vi "PID Online Autotuning (PID on the loop).vi"(0 "setpoint":dbl(slide)=30.8641975308642 scale=0.0..100.0 scale format="%.1f", 1 "manipulated variable":dbl, 3 "autotuning parameters":T2={"type of controller"=1, "relay cycles"=3, "relay amplitude"=1.0, "control specifications"=2, "PV noise level"=0.1} {"PV noise level" format="%.2f"; "control specifications" items=["Fast", "Normal", "Slow"]; "relay amplitude" format="%.2f"; "type of controller" items=["P", "PI", "PID"]}, 5 "process variable":dbl(slide)=19.583333333333336 scale=0.0..100.0 scale format="%.1f", 9 "PID gains in":T1={"proportional gain (Kc)"=1.0, "integral time (Ti, min)"=0.01, "derivative time (Td, min)"=0.0} {"derivative time (Td, min)" format="%.3f"; "integral time (Ti, min)" format="%.3f"; "proportional gain (Kc)" format="%.3f"}, 11 "dt (s)":dbl=-1.0 format="%.3f", 12 "reinitialize? (F)":bool, 13 "autotune? (F)":bool) -> (4 "setpoint out":dbl(slide)=30.8641975308642 scale=0.0..100.0 scale format="%.1f", 6 "process variable out":dbl(slide)=19.583333333333336 scale=0.0..100.0 scale format="%.1f", 8 "tuning completed?":bool, 10 "PID gains out":T1={"proportional gain (Kc)"=1.0, "integral time (Ti, min)"=0.01, "derivative time (Td, min)"=0.0} {"derivative time (Td, min)" format="%.3f"; "integral time (Ti, min)" format="%.3f"; "proportional gain (Kc)" format="%.3f"}, 14 "tuned PID gains":T1={"proportional gain (Kc)"=1.0, "integral time (Ti, min)"=0.01, "derivative time (Td, min)"=0.0} {"derivative time (Td, min)" format="%.3f"; "integral time (Ti, min)" format="%.3f"; "proportional gain (Kc)" format="%.3f"})   [LabVIEW 2020, in "NI_PID_autopid.lvlib"]
doc: "Controls the parameters of a PID controller based on the autotuning technique of the polymorphic instance you select. You can use this VI in applications with other PID VIs, such as PID or PID Advanced, to construct and tune a PID controller. You must manually select the polymorphic instance to use."
uses:
  <vilib>/addons/control/pid/NI_PID_autopid.lvlib
  <vilib>/addons/control/pid/autopid.llb/PID autotuning parameters.ctl
  <vilib>/addons/control/pid/NI_PID_pid.lvlib
panel:
  in  "Relay Setpoint":bool
  in  "Calculate Parameters":bool
  # "Relay Auto Tune"
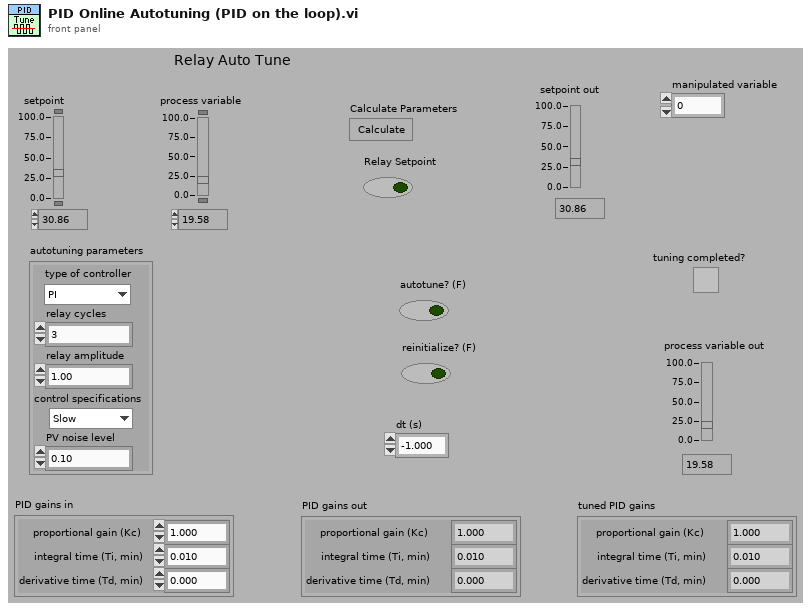
[diagram p1: front panel]
types:
  T1 = cluster{"proportional gain (Kc)":dbl, "integral time (Ti, min)":dbl, "derivative time (Td, min)":dbl}
  T2 = typedef "PID autotuning parameters.ctl" = cluster{"type of controller":u16, "relay cycles":i32, "relay amplitude":dbl, "control specifications":u16, "PV noise level":dbl}
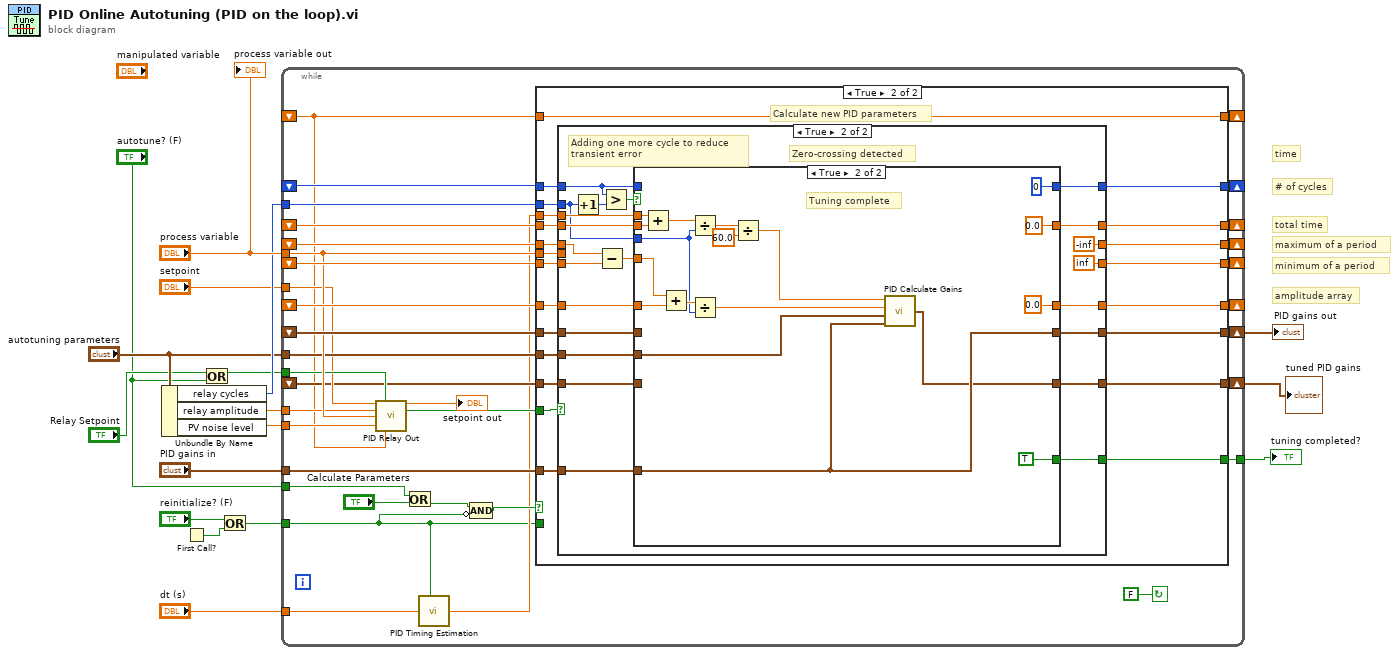
[diagram p0: block diagram]
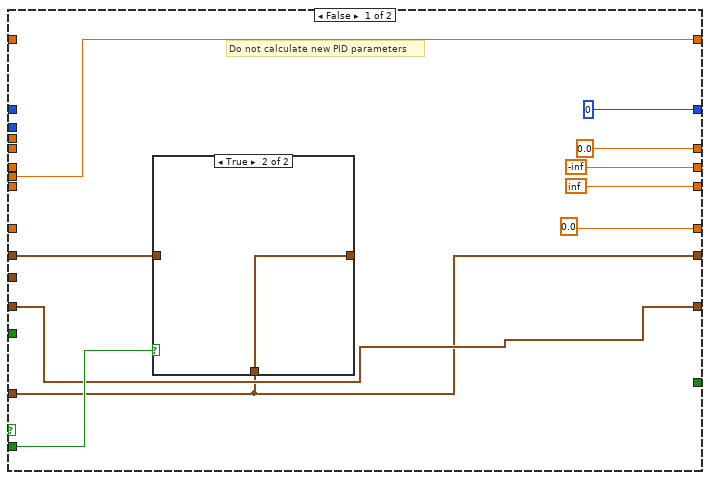
[diagram p2: hidden frame]
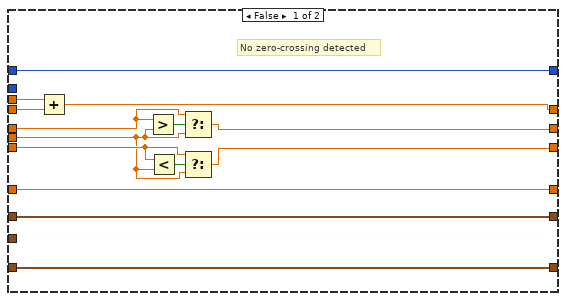
[diagram p4: hidden frame]
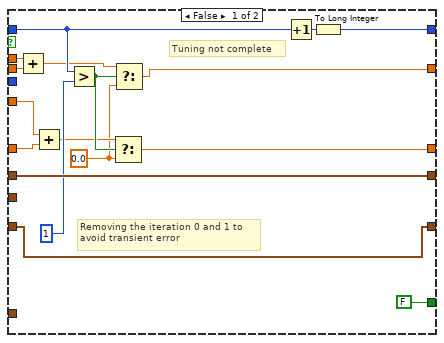
[diagram p5: hidden frame]
diagram:
  # "time"
  # "amplitude array"
  # "total time"
  # "minimum of a period"
  # "maximum of a period"
  # "# of cycles"
  n1 = Unbundle By Name("autotuning parameters") -> ("relay cycles"=w12:i32, "relay amplitude"=w8:dbl, "PV noise level"=w7:dbl)
  n2 = First Call?() -> (First Call?: T/F=w14:bool)
  n3 = Or(x="Relay Setpoint", y="autotune? (F)") -> (x .or. y?=w4:bool)
  n4 = Or(x="reinitialize? (F)", y=w14) -> (x .or. y?=w6:bool)
  n5 = while {
    shift-left: _ -> [w42]
    shift-right: [w41] -> _
    shift-left: _ -> [w44]
    shift-right: [w39] -> w17
    shift-left: _ -> [w47]
    shift-right: [w48] -> _
    shift-left: _ -> [w46]
    shift-right: [w49] -> _
    shift-left: _ -> [w50]
    shift-right: [w51] -> _
    shift-left: _ -> [w45]
    shift-right: [w52] -> _
    tunnel: w6 -> [w18]
    tunnel: "dt (s)" -> [w20]
    tunnel: "process variable" -> [w37]
    tunnel: w12 -> [w36]
    tunnel: w7 -> [w35]
    tunnel: w8 -> [w34]
    tunnel: "autotuning parameters" -> [w33]
    tunnel: "PID gains in" -> [w32]
    tunnel: "setpoint" -> [w29]
    tunnel: w4 -> [w31]
    tunnel: "autotune? (F)" -> [w28]
    shift-right: [w27] -> w2
    shift-left: _ -> [w26]
    shift-right: [w23] -> _
    shift-left: _ -> [w21]
    tunnel: [w22] -> w1
    stop <- FALSE continue-if-true
    n6 = call <vilib>:"PID Relay Out.vi"("Setpoint Reference"=w29, "Relay Setpoint"=w31, "Relay Amplitude"=w34, "Process Variable"=w37, "Noise Disturbance"=w35, "Process Variable Reference"=w21) -> ("relay output"=→"setpoint out":dbl, "Zero Crossing"=w30:bool)  [unwired: 2 in, 6 out]
    n7 = Or(x=w28, y="Calculate Parameters") -> (x .or. y?=w25:bool)
    n8 = call <vilib>:"PID Timing Estimation.vi"("Initialize?"=w18, "dt (s) in"=w20) -> ("dt (s) out"=w19:dbl)  [unwired: 7 in]
    n9 = Compound Arithmetic op=AND(w25, invert w18) -> (w24:bool)
    n10 = case shown="True" w24 {
      tunnel: w45 -> [_ w74]
      tunnel: [0 w75] -> w52
      tunnel: [-inf w76] -> w51
      tunnel: w50 -> [_ w86]
      tunnel: w46 -> [_ w85]
      tunnel: [0.0 w78] -> w49
      tunnel: [inf w77] -> w48
      tunnel: w47 -> [_ w79]
      tunnel: w36 -> [_ w83]
      tunnel: [w53 w80] -> w39
      tunnel: w44 -> [w58 w84]
      tunnel: w30 -> [_ w82]
      tunnel: w19 -> [_ w81]
      tunnel: w42 -> [_ w73]
      tunnel: [0.0 ("f") w72] -> w41
      tunnel: w33 -> [_ w71]
      tunnel: w32 -> [w53 w70]
      tunnel: w18 -> [w57 _]
      tunnel: w37 -> [w54 w69]
      tunnel: [w55 w68] -> w27
      tunnel: w26 -> [w55 w67]
      tunnel: [w54 w66] -> w23
      tunnel: w21 -> [_ w66]
      tunnel: [_ w65] -> w22
      frame False {
        # "Do not calculate new PID parameters"
        n11 = case shown="True" w57 {
          tunnel: [w63 w64] -> _
          tunnel: w58 -> [w63 _]
          tunnel: w53 -> [_ w64]
          frame False {
          }
          frame True {
          }
        }
      }
      frame True {
        # "Calculate new PID parameters"
        n12 = case shown="True" w82 {
          tunnel: w74 -> [w100 w110]
          tunnel: [w100 w112] -> w75
          tunnel: [w99 -inf] -> w76
          tunnel: w86 -> [w98 w122]
          tunnel: w85 -> [w97 w120]
          tunnel: [w97 w118] -> w78
          tunnel: [w94 inf] -> w77
          tunnel: w79 -> [w95 w121]
          tunnel: w83 -> [_ w107]
          tunnel: w84 -> [w92 w117]
          tunnel: w81 -> [w90 w116]
          tunnel: [w92 w115] -> w80
          tunnel: w73 -> [w91 w109]
          tunnel: [w89 w108] -> w72
          tunnel: w71 -> [_ w106]
          tunnel: w70 -> [_ w105]
          tunnel: w69 -> [w88 _]
          tunnel: [w87 w103] -> w68
          tunnel: w67 -> [w87 w102]
          tunnel: [_ w101] -> w65
          frame False {
            # "No zero-crossing detected"
            n13 = Add(x=w90, y=w91) -> (x+y=w89:dbl)
            n14 = Greater?(x=w98, y=w88) -> (0:w93:bool)
            n15 = Less?(x=w95, y=w88) -> (x < y?=w96:bool)
            n16 = Select(t=w98, s=w93, f=w88) -> (s? t:f=w99:dbl)
            n17 = Select(t=w95, s=w96, f=w88) -> (s? t:f=w94:dbl)
          }
          frame True {
            # "Adding one more cycle to reduce\ntransient error"
            # "Zero-crossing detected"
            n18 = Increment(x=w107) -> (x+1=w104:i32)
            n19 = Subtract(x=w122, y=w121) -> (x-y=w119:dbl)
            n20 = Greater?(x=w110, y=w104) -> (0:w111:bool)
            n21 = case shown="True" w111 {
              tunnel: w120 -> [w131 w145]
              tunnel: w119 -> [w132 w146]
              tunnel: [w126 0.0] -> w118
              tunnel: [w137 0] -> w112
              tunnel: w110 -> [w130 _]
              tunnel: [FALSE TRUE] -> w101
              tunnel: [w139 w141] -> w115
              tunnel: w117 -> [w139 _]
              tunnel: w116 -> [w136 w152]
              tunnel: w109 -> [w135 w153]
              tunnel: [w134 0.0 ("f")] -> w108
              tunnel: w107 -> [_ w143]
              tunnel: w106 -> [_ w149]
              tunnel: w105 -> [_ w141]
              tunnel: [w123 w140] -> w103
              tunnel: w102 -> [w123 _]
              frame False {
                w125 = 0.0 ("f")
                # "Removing the iteration 0 and 1 to \navoid transient error"
                # "Tuning not complete"
                n22 = Add(x=w136, y=w135) -> (x+y=w124:dbl)
                n23 = Add(x=w132, y=w131) -> (x+y=w127:dbl)
                n24 = Greater?(x=w130, y=1) -> (0:w128:bool)
                n25 = Select(t=w127, s=w128, f=w125) -> (s? t:f=w126:dbl)
                n26 = Select(t=w124, s=w128, f=w125) -> (s? t:f=w134:dbl)
                n27 = Increment(x=w130) -> (x+1=w138:i32)
                n28 = To Long Integer(number=w138) -> (32bit integer=w137:i32)
              }
              frame True {
                # "Tuning complete"
                n29 = Add(x=w152, y=w153) -> (x+y=w151:dbl)
                n30 = Add(x=w146, y=w145) -> (x+y=w144:dbl)
                n31 = Divide(x=w151, y=w143) -> (x/y=w150:dbl)
                n32 = Divide(x=w144, y=w143) -> (x/y=w142:dbl)
                n33 = Divide(x=w150, y=60.0) -> (x/y=w148:dbl)
                n34 = call <vilib>:"PID Calculate Gains.vi"("PID parameters"=w141, "autotuning parameters"=w149, "Mean amplitude"=w142, "Mean period"=w148) -> ("tuned PID parameters"=w140:cluster{"Kc":dbl, "Ti":dbl, "Td":dbl})  [unwired: 2 out]
              }
            }
          }
        }
      }
    }
  }
  "PID gains out" <- w17
  "tuned PID gains" <- w2
  "tuning completed?" <- w1
  "process variable out" <- "process variable"
